vi "MakeSpaceForControlTreminals.vi"(0 "VI Refnum":refnum<vi>, 1 "Height":i16=50, 2 "AvailableHeight":i16, 5 "error in (no error)":errorcluster) -> (19 "error out":errorcluster)   [LabVIEW 2017, in "G#IDE.lvlib" / "ScriptingLib.lvlib"]
uses:
  <resource>/Framework/Providers/AddQ/G#IDE/support/ScriptingLib/ScriptingLib.lvlib
  <vilib>/Utility/traverseref.llb/TRef TravTarget.ctl
  <vilib>/Utility/miscctls.llb/LVRectTypeDef.ctl
  <vilib>/Utility/traverseref.llb/VI Scripting - Traverse.lvlib
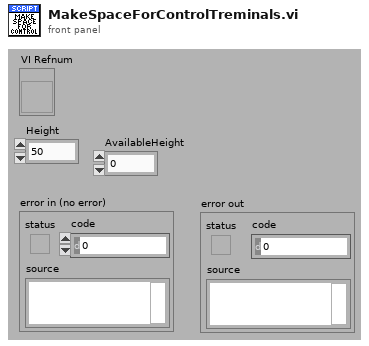
[diagram p1: front panel]
types:
  T1 = typedef "TRef TravTarget.ctl" = enum16{"FP", "BD", "Other"}
  T2 = typedef "LVRectTypeDef.ctl" = cluster{"Left":i16, "Top":i16, "Right":i16, "Bottom":i16}
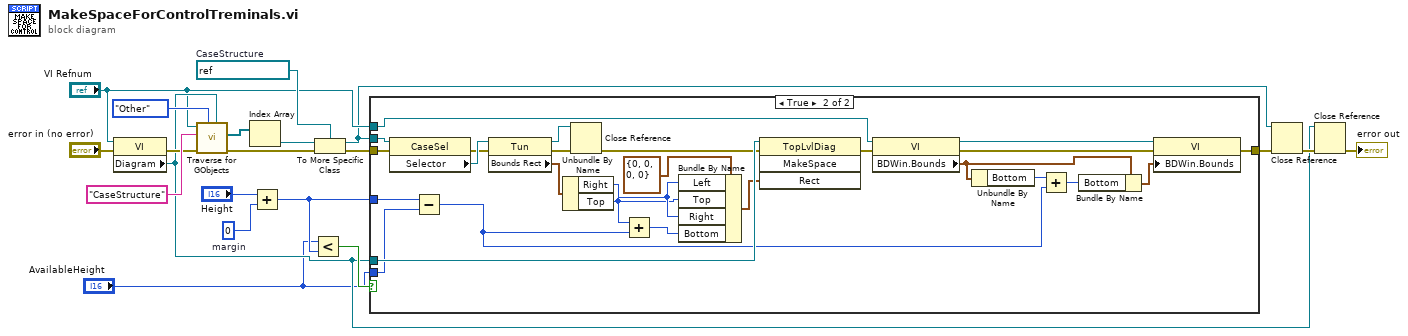
[diagram p0: block diagram]
diagram:
  w4 = i16 0  # margin
  w14 = refnum<vi> refnum  # CaseStructure
  n1 = property class="VI"(reference="VI Refnum", error in="error in (no error)") -> (error out=w18:errorcluster, "Diagram"=w6:refnum<vi>)  [unwired: 1 out]
  n2 = call <vilib>:"Traverse for GObjects.vi"("Other Refnum"=w6, "Traverse Target"=TRef_TravTarget."Other", "error in (no error)"=w18, "Class Name"="CaseStructure" ("name/order"), "VI Refnum"="VI Refnum") -> ("error out"=w15:errorcluster, "References"=w17:refnum<vi>[])  [unwired: 3 in, 2 out]
  n3 = Index Array(array=w17) -> (element=w16:refnum<vi>)  [unwired: 1 in]
  n4 = Add(x="Height", y=w4) -> (x+y=w11:i16)
  n5 = Less?(x="AvailableHeight", y=w11) -> (x < y?=w13:bool)
  n6 = To More Specific Class(target class=w14, reference=w16, error in=w15) -> (specific class reference=w2:refnum<vi>, error out=w3:errorcluster)
  n7 = case shown="True" w13 {
    tunnel: [w21 w28] -> w9
    tunnel: w6 -> [_ w46]
    tunnel: w11 -> [_ w36]
    tunnel: w3 -> [w21 w39]
    tunnel: w2 -> [_ w38]
    tunnel: "AvailableHeight" -> [_ w37]
    tunnel: "VI Refnum" -> [_ w32]
    frame False {
    }
    frame True {
      n8 = property class="CaseSel"(reference=w38, error in=w39) -> (error out=w40:errorcluster, "Selector"=w44:refnum<vi>)  [unwired: 1 out]
      n9 = Subtract(x=w36, y=w37) -> (x-y=w22:i16)
      n10 = property class="Tun"(reference=w44, error in=w40) -> (reference out=w33:refnum<vi>, error out=w35:errorcluster, "Bounds Rect"=w43:T2)
      n11 = Unbundle By Name(w43) -> ("Right"=w42:i16, "Top"=w41:i16)
      n12 = Close Reference(reference=w33, error in (no error)=w35) -> (error out=w34:errorcluster)
      n13 = Add(x=w41, y=w22) -> (x+y=w23:i16)
      n14 = Bundle By Name(cluster=T2 {"Left"=0, "Top"=0, "Right"=0, "Bottom"=0} ("Rect"), "Left"=w42, "Top"=w41, "Right"=w42, "Bottom"=w23) -> (w45:T2)
      n15 = invoke class="TopLvlDiag" method="MakeSpace"(reference=w46, error in=w34, "Rect"=w45) -> (error out=w31:errorcluster)  [unwired: 1 in, 3 out]
      n16 = property class="VI"(reference=w32, error in=w31) -> (reference out=w30:refnum<vi>, error out=w29:errorcluster, "BDWin.Bounds"=w27:T2)
      n17 = Unbundle By Name(w27) -> ("Bottom"=w25:i16)
      n18 = Add(x=w25, y=w22) -> (x+y=w24:i16)
      n19 = Bundle By Name(cluster=w27, "Bottom"=w24) -> (w26:T2)
      n20 = property class="VI"(reference=w30, error in=w29, "BDWin.Bounds"=w26) -> (error out=w28:errorcluster)  [unwired: 1 out]
    }
  }
  n21 = Close Reference(reference=w2, error in (no error)=w9) -> (error out=w8:errorcluster)
  n22 = Close Reference(reference=w6, error in (no error)=w8) -> (error out=→"error out":errorcluster)
